vi "Utility.FilterChannelsForLT.vi"(9 "DUTs":string[](array[string]), 10 "Channel":string, 11 "DUTs":bool[](array[boolean])) -> (0 "Index":i32, 3 "Use?":bool)   [LabVIEW 2015, in "TestStand Utilities.lvlib"]
uses:
  NationalInstruments.VeriStand
  TestStand Utilities.lvlib
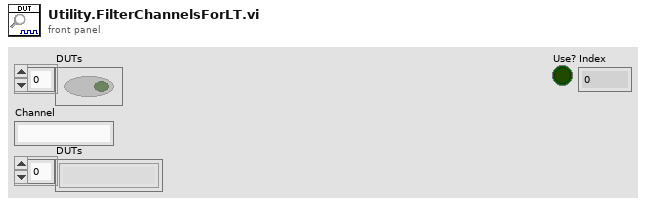
[diagram p1: front panel]
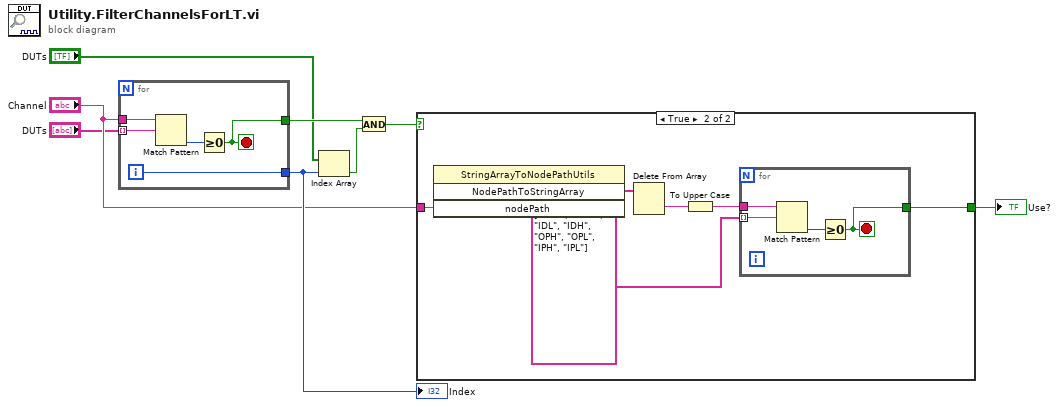
[diagram p0: block diagram]
diagram:
  n1 = for {
    tunnel: "DUTs" -> [w12] mode=indexing
    tunnel: "Channel" -> [w13]
    tunnel: [w10] -> w6
    tunnel: [w9] -> w7
    i -> [w10]
    stop <- w9 stop-if-true
    n2 = Match Pattern(string=w13, regular expression=w12) -> (offset past match=w11:i32)  [unwired: 1 in, 3 out]
    n3 = Greater Or Equal To 0?(x=w11) -> (x >= 0?=w9:bool)
  }
  "Index" <- w6
  n4 = Index Array(array="DUTs", index=w6) -> (element=w8:bool)
  n5 = And(x=w7, y=w8) -> (x .and. y?=w4:bool)
  n6 = case shown="True" w4 {
    selector: w4 -> [w14 _]
    tunnel: "Channel" -> [_ w20]
    tunnel: [w14 w15] -> w2
    frame False {
    }
    frame True {
      n7 = invoke class="StringArrayToNodePathUtils" method="NodePathToStringArray"("nodePath"=w20) -> ("NodePathToStringArray"=w19:string[])  [unwired: 3 in, 3 out]
      n8 = Delete From Array(array=w19) -> (deleted portion=w18:string)  [unwired: 2 in, 1 out]
      n9 = To Upper Case(1:w18) -> (0:w17:string)
      n10 = for {
        tunnel: string[] ["ODL", "ODH", "IDL", "IDH", "OPH", "OPL", "IPH", "IPL"] -> [w23] mode=indexing
        tunnel: w17 -> [w24]
        tunnel: [w21] -> w15
        stop <- w21 stop-if-true
        n11 = Match Pattern(string=w24, regular expression=w23) -> (offset past match=w22:i32)  [unwired: 1 in, 3 out]
        n12 = Greater Or Equal To 0?(x=w22) -> (x >= 0?=w21:bool)
      }
    }
  }
  "Use?" <- w2
